vi "Write TargetPosition.vi"(8 "error in (no error)":errorcluster, 10 "TargetPosition":i32, 11 "Picomotor8742Axis in":refnum<class "Picomotor8742Axis.lvclass">) -> (0 "error out":errorcluster, 3 "Picomotor8742Axis out":refnum<class "Picomotor8742Axis.lvclass">)   [LabVIEW 2020, in "Picomotor8742Axis.lvclass"]
uses:
  Picomotor8742Axis.lvclass
  Picomotor8742Axis.lvclass/Picomotor8742Axis.ctl
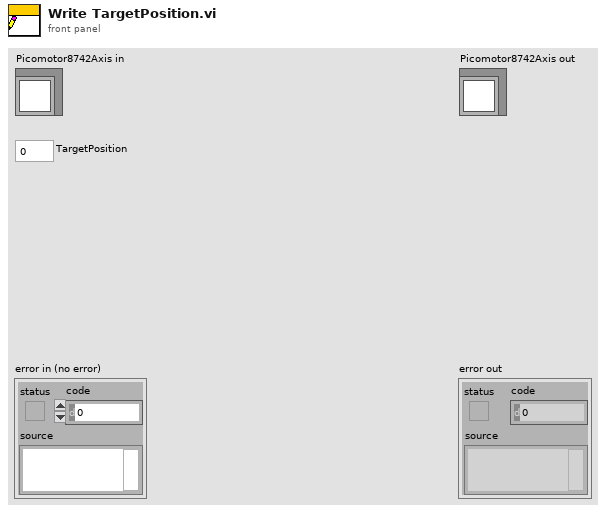
[diagram p1: front panel]
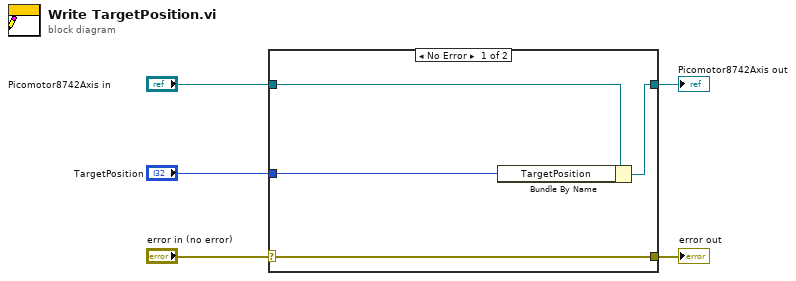
[diagram p0: block diagram]
diagram:
  n1 = case shown="No Error" "error in (no error)" {
    selector: "error in (no error)" -> [w9 w10]
    tunnel: [w9 w10] -> w4
    tunnel: [w7 w11] -> w2
    tunnel: "Picomotor8742Axis in" -> [w8 w11]
    tunnel: "TargetPosition" -> [w6 _]
    frame No Error {
      n2 = Bundle By Name(cluster=w8, "TargetPosition"=w6) -> (w7:refnum<class "Picomotor8742Axis.lvclass">)
    }
    frame Error {
    }
  }
  "error out" <- w4
  "Picomotor8742Axis out" <- w2
